vi "save Mathcad results.vi"(7 "DesignRequest":T1, 10 "error in":errorcluster, 11 "MathCAD results":T2) -> (2 "error out":errorcluster)   [LabVIEW 2012]
uses:
  Variable cluster.ctl
  Design Request.ctl
  Design Server.lvlib
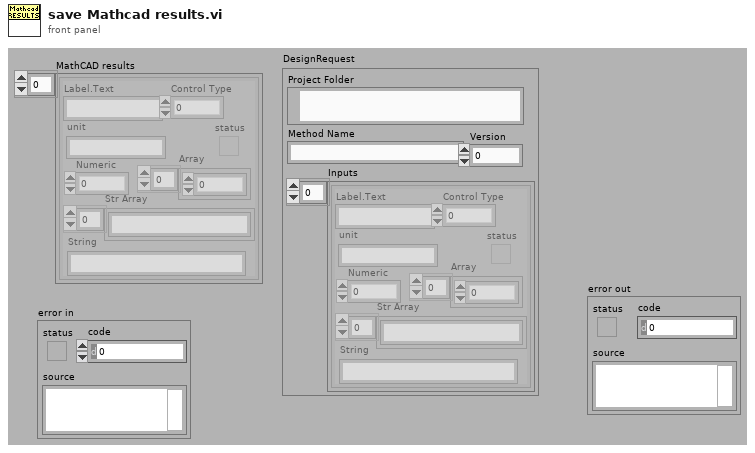
[diagram p1: front panel]
types:
  T1 = typedef "Design Server.lvlib/Design Request.ctl" = cluster{"Project Folder":path, "Method Name":string, "Inputs":T2, "Version":i32}
  T2 = typedef "Design Server.lvlib/Variable cluster.ctl" = cluster{"Label.Text":string, "Control Type":u32, "Numeric":dbl, "Array":dbl[], "status":bool, "Str Array":string[], "String":string, "unit":string}[]
  T3 = enum16{"open", "replace", "create", "open or create", "replace or create", "replace or create with confirmation"}
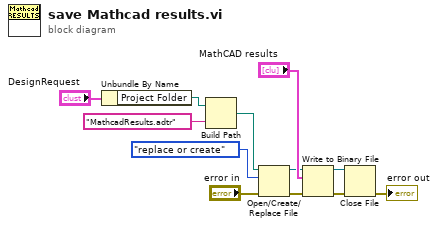
[diagram p0: block diagram]
diagram:
  n1 = Unbundle By Name("DesignRequest") -> ("Project Folder"=w5:path)
  n2 = Build Path(base path=w5, name or relative path="MathcadResults.adtr" ("File Type")) -> (appended path=w7:path)
  n3 = Open/Create/Replace File(file path (use dialog)=w7, error in="error in", operation (0:open)=T3."replace or create") -> (refnum out=w6:refnum<file>, error out=w12:errorcluster)  [unwired: 3 in, 1 out]
  n4 = Write to Binary File(file (use dialog)=w6, data="MathCAD results", error in=w12) -> (refnum out=w9:refnum<file>, error out=w10:errorcluster)  [unwired: 3 in, 1 out]
  n5 = Close File(refnum=w9, error in=w10) -> (error out=→"error out":errorcluster)  [unwired: 1 out]
